vi "Initialize RF boards - with FPGA init only vi v1.vi"(2 "error in":errorcluster, 3 "FPGA Interface":T1) -> (0 "error out":errorcluster, 1 "FPGA Interface 2":T1)   [LabVIEW 2014]
uses:
  openfpgaref.initrf.ctl
  <vilib>/Utility/error.llb/Error Cluster From Error Code.vi
  <vilib>/rvi/errors/niLvFpgaAdjustHostInterfaceError.vi
  <vilib>/rvi/interface/nirviReadWriteControl/nirviReadWriteControl.xnode
  FPGA Bitfiles/UHR-FleezersInst_FPGATarget_intitializeRFsyn_v1.lvbitx
  NiFpgaLv.dll
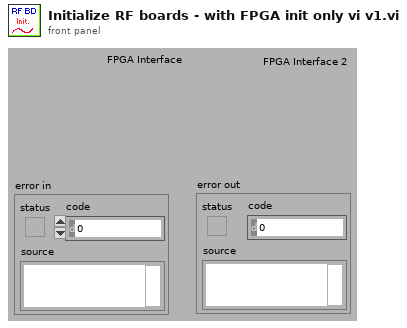
[diagram p1: front panel]
types:
  T1 = typedef "openfpgaref.initrf.ctl" = refnum<k20>
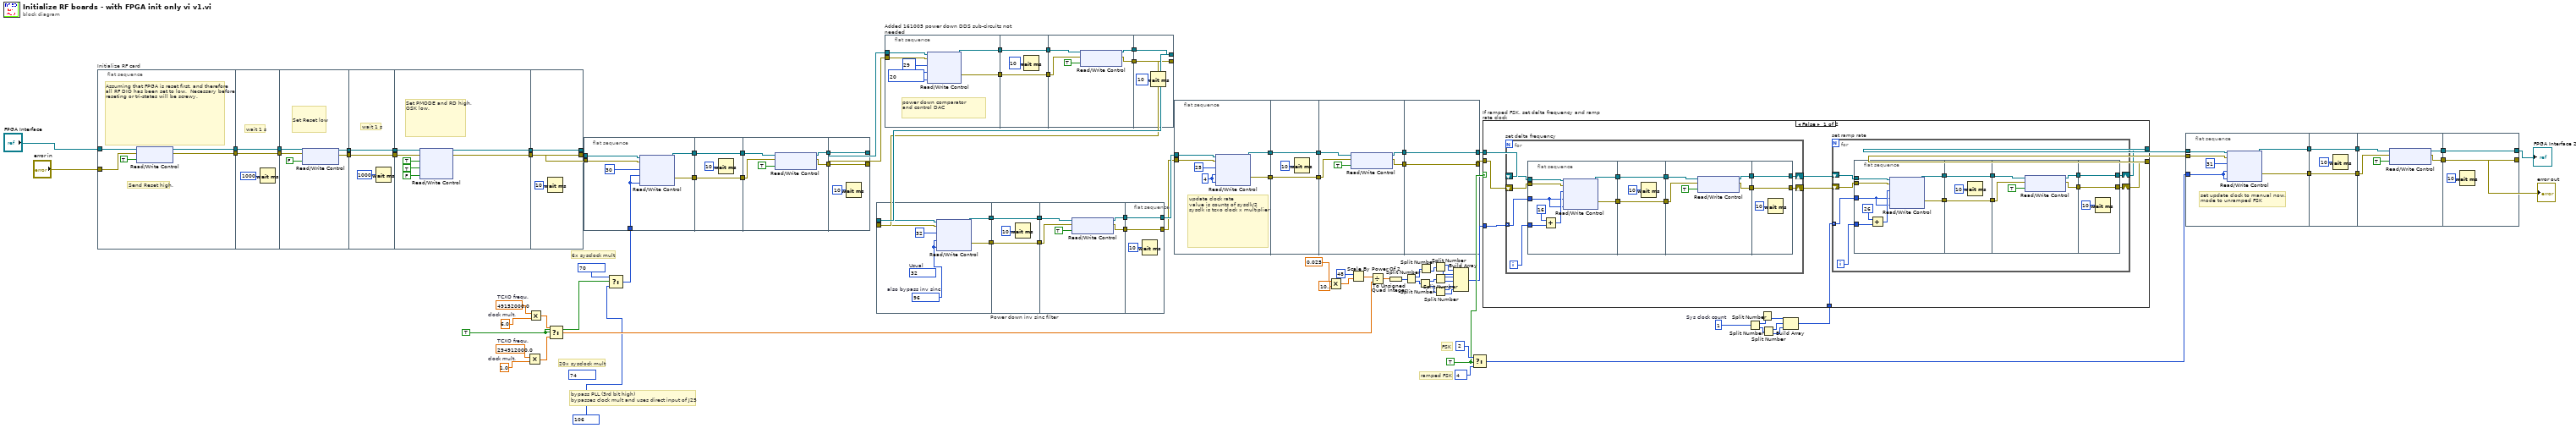
[diagram p0: block diagram]
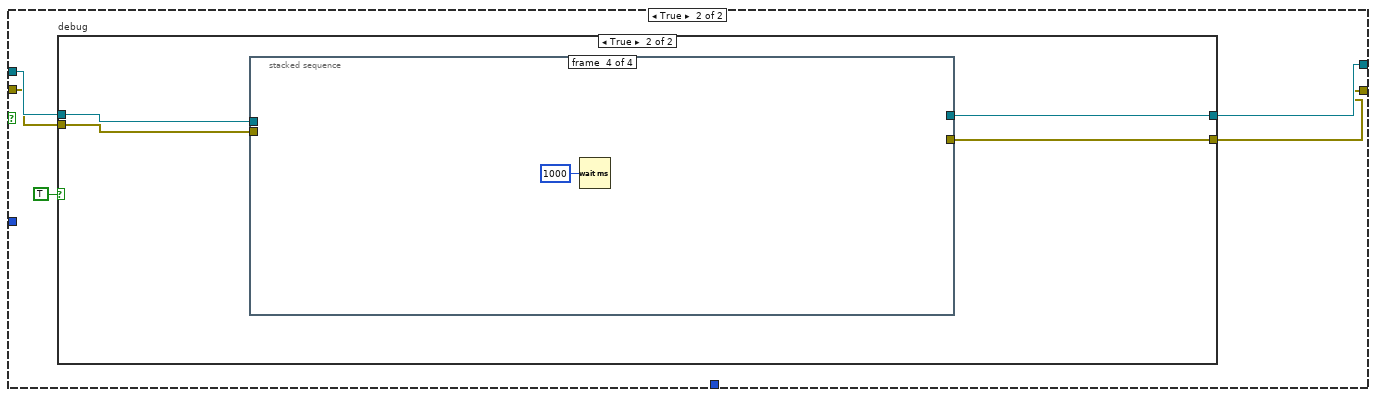
[diagram p2: hidden frame]
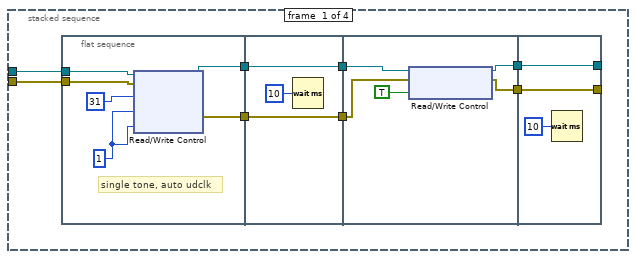
[diagram p4: hidden frame]
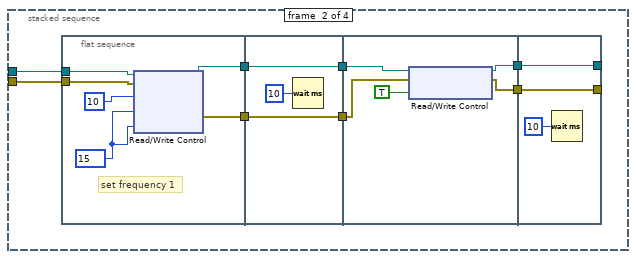
[diagram p5: hidden frame]
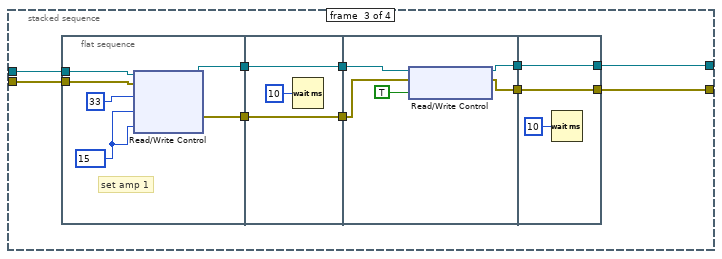
[diagram p6: hidden frame]
diagram:
  (unwired) u8 74 ("Data")
  w17 = TRUE ("s")
  w21 = 1.0  # clock mult.
  w20 = 294912000.0  # TCXO frequ.
  w24 = 6.0  # clock mult.
  w23 = 49152000.0  # TCXO frequ.
  w31 = u32 1  # Sys clock count
  w52 = TRUE
  # "bypass PLL (3rd bit high)\nbypasses clock mult and uses direct input of J25"
  # "20x sysclock mult"
  # "6x sysclock mult"
  # "ramped FSK"
  # "FSK"
  n1 = flat-sequence "Initialize RF card" {
    tunnel: [w102] -> w97
    tunnel: [w101] -> w96
    tunnel: "error in" -> [w100]
    tunnel: "FPGA Interface" -> [w98]
    tunnel: w97 -> [w104]
    tunnel: w96 -> [w103]
    tunnel: [w104] -> w95
    tunnel: [w103] -> w94
    tunnel: w95 -> [w110]
    tunnel: w94 -> [w109]
    tunnel: [w108] -> w93
    tunnel: [w107] -> w92
    tunnel: w93 -> [w112]
    tunnel: w92 -> [w111]
    tunnel: [w112] -> w91
    tunnel: [w111] -> w90
    tunnel: w91 -> [w120]
    tunnel: w90 -> [w119]
    tunnel: [w116] -> w80
    tunnel: [w115] -> w79
    tunnel: [w122] -> w73
    tunnel: [w123] -> w74
    tunnel: w80 -> [w123]
    tunnel: w79 -> [w122]
    frame #0 {
      # "Send Reset high."
      # "Assuming that FPGA is reset first, and therefore\nall RF DIO has been set to low.  Necessary before\nreseting or tri-states will be screwy."
      n2 = xnode "Read/Write Control"("FPGA VI Reference In"=w98, "error in"=w100, "Reset Bd 1"=TRUE ("Reset")) -> ("FPGA VI Reference Out"=w102:T1, "error out"=w101:errorcluster)
    }
    frame #1 {
      # "wait 1 s"
      n3 = Wait (ms)(milliseconds to wait=u32 1000) -> ()  [unwired: 1 out]
    }
    frame #2 {
      # "Set Reset low"
      n4 = xnode "Read/Write Control"("FPGA VI Reference In"=w110, "error in"=w109, "Reset Bd 1"=FALSE ("Reset")) -> ("FPGA VI Reference Out"=w108:T1, "error out"=w107:errorcluster)
    }
    frame #3 {
      # "wait 1 s"
      n5 = Wait (ms)(milliseconds to wait=u32 1000) -> ()  [unwired: 1 out]
    }
    frame #4 {
      # "Set PMODE and RD high,\nOSK low."
      n6 = xnode "Read/Write Control"("FPGA VI Reference In"=w120, "error in"=w119, "RD"=TRUE, "PMODE"=TRUE, "OSK Bd 1"=FALSE ("OSK")) -> ("FPGA VI Reference Out"=w116:T1, "error out"=w115:errorcluster)
    }
    frame #5 {
      n7 = Wait (ms)(milliseconds to wait=u32 10) -> ()  [unwired: 1 out]
    }
  }
  n8 = Multiply(x=w20, y=w21) -> (x*y=w19:dbl)
  n9 = Multiply(x=w23, y=w24) -> (x*y=w22:dbl)
  n10 = Select(t=w22, s=w17, f=w19) -> (s? t:f=w18:dbl)
  n11 = flat-sequence {
    tunnel: [w129] -> w89
    tunnel: [w128] -> w88
    tunnel: w74 -> [w127]
    tunnel: w73 -> [w126]
    tunnel: w15 -> [w124]
    tunnel: [w131] -> w87
    tunnel: w89 -> [w131]
    tunnel: [w130] -> w86
    tunnel: w88 -> [w130]
    tunnel: w87 -> [w137]
    tunnel: w86 -> [w136]
    tunnel: [w134] -> w78
    tunnel: [w133] -> w77
    tunnel: [w139] -> w6
    tunnel: [w140] -> w7
    tunnel: w78 -> [w140]
    tunnel: w77 -> [w139]
    frame #0 {
      n12 = xnode "Read/Write Control"("FPGA VI Reference In"=w127, "error in"=w126, "Address"=u8 30, "Data BD 1"=w124, "Data BD 2"=w124) -> ("FPGA VI Reference Out"=w129:T1, "error out"=w128:errorcluster)
    }
    frame #1 {
      n13 = Wait (ms)(milliseconds to wait=u32 10) -> ()  [unwired: 1 out]
    }
    frame #2 {
      n14 = xnode "Read/Write Control"("FPGA VI Reference In"=w137, "error in"=w136, "Update Data"=TRUE) -> ("FPGA VI Reference Out"=w134:T1, "error out"=w133:errorcluster)
    }
    frame #3 {
      n15 = Wait (ms)(milliseconds to wait=u32 10) -> ()  [unwired: 1 out]
    }
  }
  n16 = Select(t=u8 70 ("Data"), s=w17, f=u8 106 ("Data")) -> (s? t:f=w15:u8)
  n17 = flat-sequence "Power down inv sinc filter" {
    tunnel: [w146] -> w85
    tunnel: [w145] -> w84
    tunnel: w5 -> [w144]
    tunnel: w4 -> [w143]
    tunnel: [w148] -> w83
    tunnel: w85 -> [w148]
    tunnel: [w147] -> w82
    tunnel: w84 -> [w147]
    tunnel: w83 -> [w154]
    tunnel: w82 -> [w153]
    tunnel: [w151] -> w76
    tunnel: [w150] -> w75
    tunnel: [w156] -> w65
    tunnel: [w157] -> w66
    tunnel: w76 -> [w157]
    tunnel: w75 -> [w156]
    frame #0 {
      w141 = u8 96  # also bypass inv sinc
      (unwired) u8 32  # Usual
      n18 = xnode "Read/Write Control"("FPGA VI Reference In"=w144, "error in"=w143, "Address"=u8 32, "Data BD 1"=w141, "Data BD 2"=w141) -> ("FPGA VI Reference Out"=w146:T1, "error out"=w145:errorcluster)
    }
    frame #1 {
      n19 = Wait (ms)(milliseconds to wait=u32 10) -> ()  [unwired: 1 out]
    }
    frame #2 {
      n20 = xnode "Read/Write Control"("FPGA VI Reference In"=w154, "error in"=w153, "Update Data"=TRUE) -> ("FPGA VI Reference Out"=w151:T1, "error out"=w150:errorcluster)
    }
    frame #3 {
      n21 = Wait (ms)(milliseconds to wait=u32 10) -> ()  [unwired: 1 out]
    }
  }
  n22 = flat-sequence "Added 161005 power down DDS sub-circuits not needed" {
    tunnel: [w163] -> w13
    tunnel: [w162] -> w12
    tunnel: w7 -> [w161]
    tunnel: w6 -> [w160]
    tunnel: [w165] -> w11
    tunnel: w13 -> [w165]
    tunnel: [w164] -> w10
    tunnel: w12 -> [w164]
    tunnel: w11 -> [w171]
    tunnel: w10 -> [w170]
    tunnel: [w168] -> w9
    tunnel: [w167] -> w8
    tunnel: [w174] -> w4
    tunnel: w9 -> [w172]
    tunnel: w8 -> [w174]
    tunnel: [w172] -> w5
    frame #0 {
      w158 = u8 20 ("Data")
      # "power down comparator\nand control DAC"
      n23 = xnode "Read/Write Control"("FPGA VI Reference In"=w161, "error in"=w160, "Address"=u8 29, "Data BD 1"=w158, "Data BD 2"=w158) -> ("FPGA VI Reference Out"=w163:T1, "error out"=w162:errorcluster)
    }
    frame #1 {
      n24 = Wait (ms)(milliseconds to wait=u32 10) -> ()  [unwired: 1 out]
    }
    frame #2 {
      n25 = xnode "Read/Write Control"("FPGA VI Reference In"=w171, "error in"=w170, "Update Data"=TRUE) -> ("FPGA VI Reference Out"=w168:T1, "error out"=w167:errorcluster)
    }
    frame #3 {
      n26 = Wait (ms)(milliseconds to wait=u32 10) -> ()  [unwired: 1 out]
    }
  }
  n27 = flat-sequence {
    tunnel: [w180] -> w72
    tunnel: [w179] -> w71
    tunnel: w66 -> [w178]
    tunnel: w65 -> [w177]
    tunnel: [w182] -> w70
    tunnel: w72 -> [w182]
    tunnel: [w181] -> w69
    tunnel: w71 -> [w181]
    tunnel: w70 -> [w188]
    tunnel: w69 -> [w187]
    tunnel: [w185] -> w68
    tunnel: [w184] -> w67
    tunnel: [w189] -> w63
    tunnel: [w190] -> w64
    tunnel: w68 -> [w190]
    tunnel: w67 -> [w189]
    frame #0 {
      w175 = u8 4 ("Data")
      # "update clock rate\nvalue is counts of sysclk/2\nsysclk is tcxo clock x multiplier"
      n28 = xnode "Read/Write Control"("FPGA VI Reference In"=w178, "error in"=w177, "Address"=u8 25, "Data BD 1"=w175, "Data BD 2"=w175) -> ("FPGA VI Reference Out"=w180:T1, "error out"=w179:errorcluster)
    }
    frame #1 {
      n29 = Wait (ms)(milliseconds to wait=u32 10) -> ()  [unwired: 1 out]
    }
    frame #2 {
      n30 = xnode "Read/Write Control"("FPGA VI Reference In"=w188, "error in"=w187, "Update Data"=TRUE) -> ("FPGA VI Reference Out"=w185:T1, "error out"=w184:errorcluster)
    }
    frame #3 {
    }
  }
  n31 = Multiply(x=0.025 ("Delta Frequency  (MHz)"), y=1000000.0) -> (x*y=w47:dbl)
  n32 = Scale By Power Of 2(n=48, x=w47) -> (x*2^n=w49:dbl)
  n33 = Divide(x=w49, y=w18) -> (x/y=w48:dbl)
  n34 = To Unsigned Quad Integer(1:w48) -> (0:w44:u64)
  n35 = Split Number(x=w44) -> (hi(x)=w43:u32, lo(x)=w42:u32)
  n36 = Split Number(x=w42) -> (hi(x)=w40:u16, lo(x)=w41:u16)
  n37 = Split Number(x=w43) -> (lo(x)=w39:u16)  [unwired: 1 out]
  n38 = Split Number(x=w39) -> (hi(x)=w38:u8, lo(x)=w37:u8)
  n39 = Split Number(x=w40) -> (hi(x)=w36:u8, lo(x)=w35:u8)
  n40 = Split Number(x=w41) -> (hi(x)=w34:u8, lo(x)=w33:u8)
  n41 = Build Array(w38, w37, w36, w35, w34, w33) -> (w32:u8[])
  n42 = Select(t=u8 2 ("Data"), s=w52, f=u8 4 ("Data")) -> (s? t:f=w53:u8)
  n43 = Split Number(x=w31) -> (hi(x)=w30:u16, lo(x)=w29:u16)
  n44 = Split Number(x=w30) -> (lo(x)=w28:u8)  [unwired: 1 out]
  n45 = Split Number(x=w29) -> (hi(x)=w27:u8, lo(x)=w26:u8)
  n46 = Build Array(w28, w27, w26) -> (w25:u8[])
  n47 = case "If ramped FSK, set delta frequency and ramp rate clock" shown="False" w52 {
    tunnel: w64 -> [w198 w265]
    tunnel: w63 -> [w197 w264]
    tunnel: [w192 w261] -> w60
    tunnel: [w193 w262] -> w59
    tunnel: w32 -> [w196 _]
    tunnel: w25 -> [w191 _]
    frame False {
      n48 = for "set delta frequency" {
        shift-right: [w232] -> w195
        shift-left: w198 -> [w235]
        shift-right: [w233] -> w194
        shift-left: w197 -> [w234]
        tunnel: w196 -> [w230] mode=indexing
        i -> [w231]
        n49 = flat-sequence {
          tunnel: [w249] -> w241
          tunnel: [w248] -> w240
          tunnel: w235 -> [w247]
          tunnel: w234 -> [w246]
          tunnel: w231 -> [w244]
          tunnel: w230 -> [w242]
          tunnel: [w251] -> w239
          tunnel: w241 -> [w251]
          tunnel: [w250] -> w238
          tunnel: w240 -> [w250]
          tunnel: w239 -> [w257]
          tunnel: w238 -> [w256]
          tunnel: [w254] -> w237
          tunnel: [w253] -> w236
          tunnel: [w260] -> w233
          tunnel: [w258] -> w232
          tunnel: w237 -> [w258]
          tunnel: w236 -> [w260]
          frame #0 {
            n50 = Add(x=u8 16 ("Address"), y=w244) -> (x+y=w243:i32)
            n51 = xnode "Read/Write Control"("FPGA VI Reference In"=w247, "error in"=w246, "Address"=w243, "Data BD 1"=w242, "Data BD 2"=w242) -> ("FPGA VI Reference Out"=w249:T1, "error out"=w248:errorcluster)
          }
          frame #1 {
            n52 = Wait (ms)(milliseconds to wait=u32 10) -> ()  [unwired: 1 out]
          }
          frame #2 {
            n53 = xnode "Read/Write Control"("FPGA VI Reference In"=w257, "error in"=w256, "Update Data"=TRUE) -> ("FPGA VI Reference Out"=w254:T1, "error out"=w253:errorcluster)
          }
          frame #3 {
            n54 = Wait (ms)(milliseconds to wait=u32 10) -> ()  [unwired: 1 out]
          }
        }
      }
      n55 = for "set ramp rate" {
        shift-right: [w201] -> w193
        shift-left: w195 -> [w204]
        shift-right: [w202] -> w192
        shift-left: w194 -> [w203]
        tunnel: w191 -> [w199] mode=indexing
        i -> [w200]
        n56 = flat-sequence {
          tunnel: [w218] -> w210
          tunnel: [w217] -> w209
          tunnel: w204 -> [w216]
          tunnel: w203 -> [w215]
          tunnel: w200 -> [w213]
          tunnel: w199 -> [w211]
          tunnel: [w220] -> w208
          tunnel: w210 -> [w220]
          tunnel: [w219] -> w207
          tunnel: w209 -> [w219]
          tunnel: w208 -> [w226]
          tunnel: w207 -> [w225]
          tunnel: [w223] -> w206
          tunnel: [w222] -> w205
          tunnel: [w229] -> w202
          tunnel: [w227] -> w201
          tunnel: w206 -> [w227]
          tunnel: w205 -> [w229]
          frame #0 {
            n57 = Add(x=u8 26 ("Address"), y=w213) -> (x+y=w212:i32)
            n58 = xnode "Read/Write Control"("FPGA VI Reference In"=w216, "error in"=w215, "Address"=w212, "Data BD 1"=w211, "Data BD 2"=w211) -> ("FPGA VI Reference Out"=w218:T1, "error out"=w217:errorcluster)
          }
          frame #1 {
            n59 = Wait (ms)(milliseconds to wait=u32 10) -> ()  [unwired: 1 out]
          }
          frame #2 {
            n60 = xnode "Read/Write Control"("FPGA VI Reference In"=w226, "error in"=w225, "Update Data"=TRUE) -> ("FPGA VI Reference Out"=w223:T1, "error out"=w222:errorcluster)
          }
          frame #3 {
            n61 = Wait (ms)(milliseconds to wait=u32 10) -> ()  [unwired: 1 out]
          }
        }
      }
    }
    frame True {
      n62 = case "debug" shown="True" TRUE {
        tunnel: w265 -> [w267 w271]
        tunnel: w264 -> [w266 w270]
        tunnel: [w267 w269] -> w262
        tunnel: [w266 w268] -> w261
        frame False {
        }
        frame True {
          n63 = stacked-sequence {
            tunnel: w271 -> [w273 w298 w325 _]
            tunnel: w270 -> [w272 w297 w324 _]
            tunnel: [_ _ w323 _] -> w269
            tunnel: [_ _ w322 _] -> w268
            frame #0 {
              n64 = flat-sequence {
                tunnel: [w285] -> w279
                tunnel: [w284] -> w278
                tunnel: w273 -> [w283]
                tunnel: w272 -> [w282]
                tunnel: [w287] -> w277
                tunnel: w279 -> [w287]
                tunnel: [w286] -> w276
                tunnel: w278 -> [w286]
                tunnel: w277 -> [w293]
                tunnel: w276 -> [w292]
                tunnel: [w290] -> w275
                tunnel: [w289] -> w274
                tunnel: [w296] -> _
                tunnel: [w294] -> _
                tunnel: w275 -> [w294]
                tunnel: w274 -> [w296]
                frame #0 {
                  w280 = u8 1 ("Data")
                  # "single tone, auto udclk"
                  n65 = xnode "Read/Write Control"("FPGA VI Reference In"=w283, "error in"=w282, "Address"=u8 31, "Data BD 1"=w280, "Data BD 2"=w280) -> ("FPGA VI Reference Out"=w285:T1, "error out"=w284:errorcluster)
                }
                frame #1 {
                  n66 = Wait (ms)(milliseconds to wait=u32 10) -> ()  [unwired: 1 out]
                }
                frame #2 {
                  n67 = xnode "Read/Write Control"("FPGA VI Reference In"=w293, "error in"=w292, "Update Data"=TRUE) -> ("FPGA VI Reference Out"=w290:T1, "error out"=w289:errorcluster)
                }
                frame #3 {
                  n68 = Wait (ms)(milliseconds to wait=u32 10) -> ()  [unwired: 1 out]
                }
              }
            }
            frame #1 {
              n69 = flat-sequence {
                tunnel: [w310] -> w304
                tunnel: [w309] -> w303
                tunnel: w298 -> [w308]
                tunnel: w297 -> [w307]
                tunnel: [w312] -> w302
                tunnel: w304 -> [w312]
                tunnel: [w311] -> w301
                tunnel: w303 -> [w311]
                tunnel: w302 -> [w318]
                tunnel: w301 -> [w317]
                tunnel: [w315] -> w300
                tunnel: [w314] -> w299
                tunnel: [w321] -> _
                tunnel: [w319] -> _
                tunnel: w300 -> [w319]
                tunnel: w299 -> [w321]
                frame #0 {
                  w305 = u8 15 ("Data")
                  # "set frequency 1"
                  n70 = xnode "Read/Write Control"("FPGA VI Reference In"=w308, "error in"=w307, "Address"=u8 10, "Data BD 1"=w305, "Data BD 2"=w305) -> ("FPGA VI Reference Out"=w310:T1, "error out"=w309:errorcluster)
                }
                frame #1 {
                  n71 = Wait (ms)(milliseconds to wait=u32 10) -> ()  [unwired: 1 out]
                }
                frame #2 {
                  n72 = xnode "Read/Write Control"("FPGA VI Reference In"=w318, "error in"=w317, "Update Data"=TRUE) -> ("FPGA VI Reference Out"=w315:T1, "error out"=w314:errorcluster)
                }
                frame #3 {
                  n73 = Wait (ms)(milliseconds to wait=u32 10) -> ()  [unwired: 1 out]
                }
              }
            }
            frame #2 {
              n74 = flat-sequence {
                tunnel: [w337] -> w331
                tunnel: [w336] -> w330
                tunnel: w325 -> [w335]
                tunnel: w324 -> [w334]
                tunnel: [w339] -> w329
                tunnel: w331 -> [w339]
                tunnel: [w338] -> w328
                tunnel: w330 -> [w338]
                tunnel: w329 -> [w345]
                tunnel: w328 -> [w344]
                tunnel: [w342] -> w327
                tunnel: [w341] -> w326
                tunnel: [w348] -> w322
                tunnel: [w346] -> w323
                tunnel: w327 -> [w346]
                tunnel: w326 -> [w348]
                frame #0 {
                  w332 = u8 15 ("Data")
                  # "set amp 1"
                  n75 = xnode "Read/Write Control"("FPGA VI Reference In"=w335, "error in"=w334, "Address"=u8 33, "Data BD 1"=w332, "Data BD 2"=w332) -> ("FPGA VI Reference Out"=w337:T1, "error out"=w336:errorcluster)
                }
                frame #1 {
                  n76 = Wait (ms)(milliseconds to wait=u32 10) -> ()  [unwired: 1 out]
                }
                frame #2 {
                  n77 = xnode "Read/Write Control"("FPGA VI Reference In"=w345, "error in"=w344, "Update Data"=TRUE) -> ("FPGA VI Reference Out"=w342:T1, "error out"=w341:errorcluster)
                }
                frame #3 {
                  n78 = Wait (ms)(milliseconds to wait=u32 10) -> ()  [unwired: 1 out]
                }
              }
            }
            frame #3 {
              n79 = Wait (ms)(milliseconds to wait=u32 1000) -> ()  [unwired: 1 out]
            }
          }
        }
      }
    }
  }
  n80 = flat-sequence {
    tunnel: [w355] -> w58
    tunnel: [w354] -> w57
    tunnel: w59 -> [w353]
    tunnel: w60 -> [w352]
    tunnel: w53 -> [w350]
    tunnel: [w357] -> w56
    tunnel: w58 -> [w357]
    tunnel: [w356] -> w55
    tunnel: w57 -> [w356]
    tunnel: w56 -> [w363]
    tunnel: w55 -> [w362]
    tunnel: [w360] -> w54
    tunnel: [w359] -> w2
    tunnel: [w366] -> w51
    tunnel: w54 -> [w366]
    tunnel: [w364] -> w1
    tunnel: w2 -> [w364]
    frame #0 {
      # "set update clock to manual now,\nmode to unramped FSK"
      n81 = xnode "Read/Write Control"("FPGA VI Reference In"=w353, "error in"=w352, "Address"=u8 31, "Data BD 1"=w350, "Data BD 2"=w350) -> ("FPGA VI Reference Out"=w355:T1, "error out"=w354:errorcluster)
    }
    frame #1 {
      n82 = Wait (ms)(milliseconds to wait=u32 10) -> ()  [unwired: 1 out]
    }
    frame #2 {
      n83 = xnode "Read/Write Control"("FPGA VI Reference In"=w363, "error in"=w362, "Update Data"=TRUE) -> ("FPGA VI Reference Out"=w359:T1, "error out"=w360:errorcluster)
    }
    frame #3 {
      n84 = Wait (ms)(milliseconds to wait=u32 10) -> ()  [unwired: 1 out]
    }
  }
  "error out" <- w51
  "FPGA Interface 2" <- w1
